vi "LoadFileNew.vi"(11 "folder":string="QAMT01\\CRH3605") -> (1 "f":bool, 3 "Lot":string)   [LabVIEW 2012]
uses:
  Global1.vi
panel:
  out "text":string
  out "before substring":string
  out "after substring":string
  out "String":string
  out "error out":errorcluster
  in  "error in (no error)":errorcluster
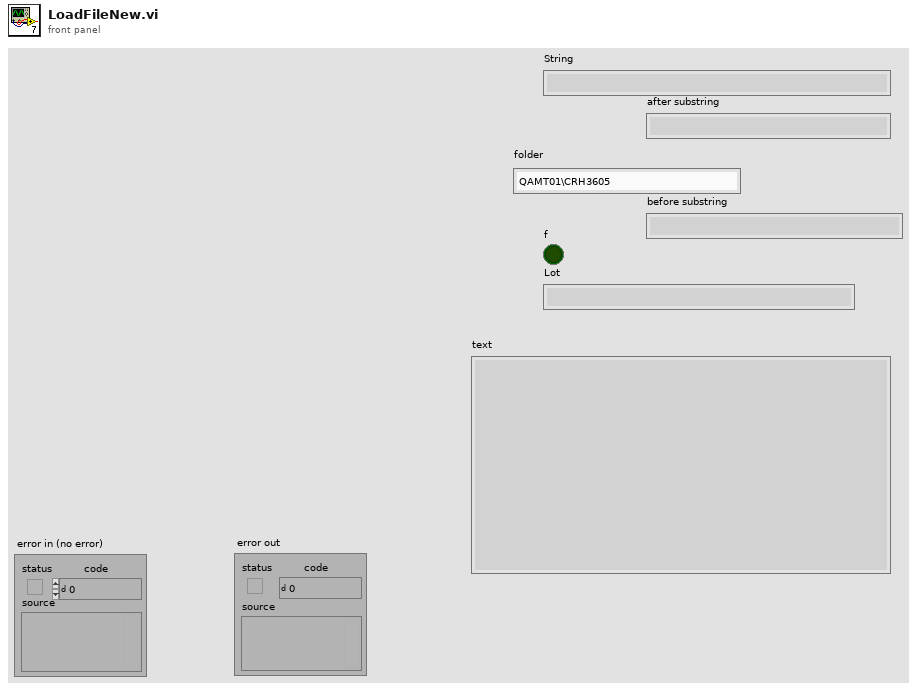
[diagram p1: front panel]
types:
  T1 = enum16{"open", "replace", "create", "open or create", "replace or create", "replace or create with confirmation"}
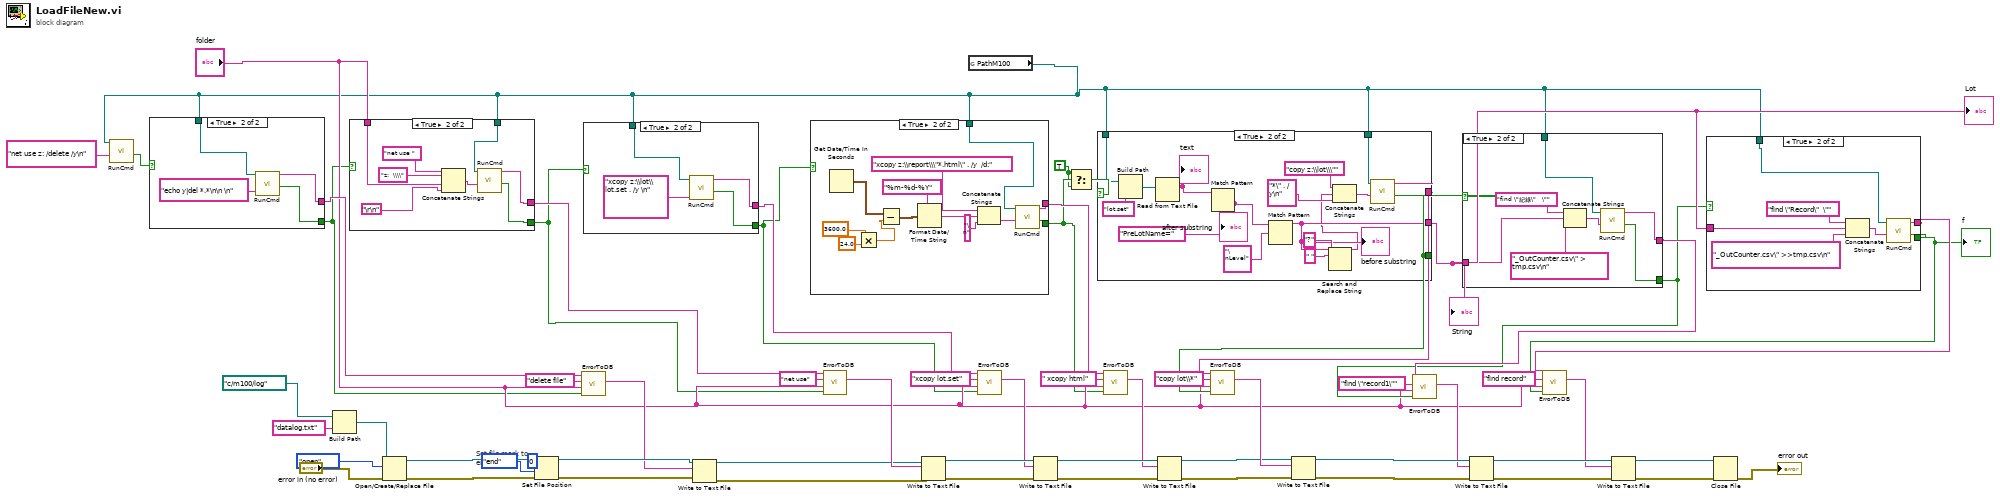
[diagram p0: block diagram]
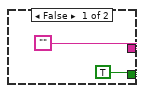
[diagram p2: hidden frame]
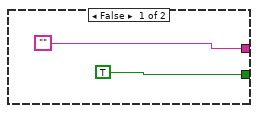
[diagram p3: hidden frame]
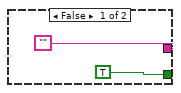
[diagram p4: hidden frame]
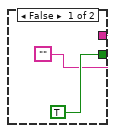
[diagram p5: hidden frame]
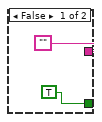
[diagram p6: hidden frame]
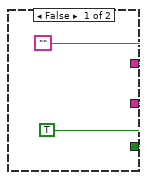
[diagram p7: hidden frame]
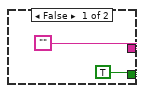
[diagram p8: hidden frame]
diagram:
  w6 = TRUE
  # "Set file mark to\nend of file"
  n1 = Build Path(base path=path "c:/m100/log", name or relative path="datalog.txt") -> (appended path=w53:path)
  n2 = Open/Create/Replace File(file path (use dialog)=w53, error in="error in (no error)", operation (0:open)=T1."open") -> (refnum out=w58:refnum<file>, error out=w57:errorcluster)  [unwired: 3 in, 1 out]
  n3 = Set File Position(offset (in bytes) (0)=i64 0, refnum=w58, from (0:start)=enum16{"start", "end", "current"}."end", error in=w57) -> (refnum out=w22:refnum<file>, error out=w21:errorcluster)
  n4 = global read "Global1.vi" "PathM100"() -> (w5:path)
  n5 = call "RunCmd.vi"("Cmd String"="net use z: /delete /y\n" ("string"), "working directory"=w5) -> ("OK"=w23:bool)  [unwired: 8 in, 1 out]
  n6 = case shown="True" w23 {
    tunnel: [TRUE w65] -> w3
    tunnel: ["" w64] -> w18
    tunnel: w5 -> [_ w67]
    frame False {
    }
    frame True {
      n7 = call "RunCmd.vi"("Cmd String"="echo y|del *.*\n\n \n" ("standard input"), "working directory"=w67) -> ("OK"=w65:bool, "Output"=w64:string)  [unwired: 8 in]
    }
  }
  n8 = case shown="True" w3 {
    tunnel: [TRUE w70] -> w4
    tunnel: ["" w71] -> w31
    tunnel: "folder" -> [_ w73]
    tunnel: w5 -> [_ w72]
    frame False {
    }
    frame True {
      n9 = Concatenate Strings("net use " ("string"), "z:  \\\\" ("string"), w73, "\r\n") -> (w77:string)
      n10 = call "RunCmd.vi"("Cmd String"=w77, "working directory"=w72) -> ("OK"=w70:bool, "Output"=w71:string)  [unwired: 8 in]
    }
  }
  n11 = call "ErrorToDB.vi"("Error"=w3, "Folder"="folder", "Command"="delete file", "Error Message"=w18) -> ("LogData"=w17:string)  [unwired: 7 in]
  n12 = case shown="True" w4 {
    tunnel: [TRUE w81] -> w2
    tunnel: ["" w80] -> w30
    tunnel: w5 -> [_ w83]
    frame False {
    }
    frame True {
      n13 = call "RunCmd.vi"("Cmd String"="xcopy z:\\lot\\lot.set . /y \n" ("standard input"), "working directory"=w83) -> ("OK"=w81:bool, "Output"=w80:string)  [unwired: 8 in]
    }
  }
  n14 = Write to Text File(file (use dialog)=w22, text=w17, error in=w21) -> (refnum out=w20:refnum<file>, error out=w19:errorcluster)  [unwired: 1 in, 1 out]
  n15 = case shown="True" w2 {
    tunnel: [TRUE w87] -> w8
    tunnel: ["" w88] -> w29
    tunnel: w5 -> [_ w86]
    frame False {
    }
    frame True {
      n16 = Get Date/Time In Seconds() -> (seconds since 1Jan1904=w89:timestamp)
      n17 = Multiply(x=3600.0, y=24.0) -> (x*y=w91:dbl)
      n18 = Subtract(x=w89, y=w91) -> (x-y=w92:timestamp)
      n19 = Format Date/Time String(time format string (%c)="%m-%d-%Y", seconds (now)=w92) -> (date/time string=w95:string)  [unwired: 1 in]
      n20 = Concatenate Strings("xcopy z:\\report\\\"*.html\" . /y  /d:" ("string"), w95, "\n" ("string")) -> (w98:string)
      n21 = call "RunCmd.vi"("Cmd String"=w98, "working directory"=w86) -> ("OK"=w87:bool, "Output"=w88:string)  [unwired: 8 in]
    }
  }
  n22 = call "ErrorToDB.vi"("Error"=w4, "Folder"="folder", "Command"="net use", "Error Message"=w31) -> ("LogData"=w43:string)  [unwired: 7 in]
  n23 = Write to Text File(file (use dialog)=w20, text=w43, error in=w19) -> (refnum out=w52:refnum<file>, error out=w51:errorcluster)  [unwired: 1 in, 1 out]
  n24 = call "ErrorToDB.vi"("Error"=w2, "Folder"="folder", "Command"="xcopy lot.set", "Error Message"=w30) -> ("LogData"=w42:string)  [unwired: 7 in]
  n25 = Write to Text File(file (use dialog)=w52, text=w42, error in=w51) -> (refnum out=w28:refnum<file>, error out=w27:errorcluster)  [unwired: 1 in, 1 out]
  n26 = Select(t=w6, s=w8, f=w6) -> (s? t:f=w7:bool)
  n27 = case shown="True" w7 {
    tunnel: [TRUE w105] -> w38
    tunnel: [w99 w106] -> w39
    tunnel: w5 -> [_ w109]
    tunnel: [w99 w102] -> w44
    tunnel: w5 -> [_ w107]
    frame False {
      w99 = ""
    }
    frame True {
      n28 = Build Path(base path=w109, name or relative path="lot.set") -> (appended path=w117:path)
      n29 = Read from Text File(file (use dialog)=w117) -> (text=w114:string)  [unwired: 3 in, 3 out]
      "text" <- w114
      n30 = Match Pattern(string=w114, regular expression="PreLotName=") -> (after substring=w110:string)  [unwired: 1 in, 3 out]
      "after substring" <- w110
      n31 = Match Pattern(string=w110, regular expression="\nLevel") -> (before substring=w102:string)  [unwired: 1 in, 3 out]
      "before substring" <- w102
      n32 = Search and Replace String(input string=w102, search string=" ", replace string="?" ("replace string (\"\")")) -> (result string=w101:string)  [unwired: 5 in, 3 out]
      n33 = Concatenate Strings("copy z:\\lot\\\"" ("string"), w101, "*\" . /y\n" ("string")) -> (w108:string)
      n34 = call "RunCmd.vi"("Cmd String"=w108, "working directory"=w107) -> ("OK"=w105:bool, "Output"=w106:string)  [unwired: 8 in]
    }
  }
  "Lot" <- w44
  "String" <- w44
  n35 = call "ErrorToDB.vi"("Error"=w8, "Folder"="folder", "Command"=" xcopy html", "Error Message"=w29) -> ("LogData"=w24:string)  [unwired: 7 in]
  n36 = Write to Text File(file (use dialog)=w28, text=w24, error in=w27) -> (refnum out=w26:refnum<file>, error out=w25:errorcluster)  [unwired: 1 in, 1 out]
  n37 = call "ErrorToDB.vi"("Error"=w38, "Folder"="folder", "Command"="copy lot\\*", "Error Message"=w39) -> ("LogData"=w40:string)  [unwired: 7 in]
  n38 = Write to Text File(file (use dialog)=w26, text=w40, error in=w25) -> (refnum out=w50:refnum<file>, error out=w49:errorcluster)  [unwired: 1 in, 1 out]
  n39 = case shown="True" w38 {
    tunnel: ["" w121] -> w36
    tunnel: w44 -> [_ w125]
    tunnel: w5 -> [_ w122]
    tunnel: [TRUE w120] -> w35
    frame False {
    }
    frame True {
      n40 = Concatenate Strings("find \"紀錄\"   \"" ("string"), w125, "_OutCounter.csv\" > tmp.csv\n" ("string")) -> (w123:string)
      n41 = call "RunCmd.vi"("Cmd String"=w123, "working directory"=w122) -> ("OK"=w120:bool, "Output"=w121:string)  [unwired: 8 in]
    }
  }
  n42 = call "ErrorToDB.vi"("Error"=w35, "Folder"="folder", "Command"="find \"record1\"", "Error Message"=w36) -> ("LogData"=w37:string)  [unwired: 7 in]
  n43 = Write to Text File(file (use dialog)=w50, text=w37, error in=w49) -> (refnum out=w48:refnum<file>, error out=w46:errorcluster)  [unwired: 1 in, 1 out]
  n44 = case shown="True" w35 {
    tunnel: w5 -> [_ w132]
    tunnel: w44 -> [_ w133]
    tunnel: ["" w129] -> w33
    tunnel: [TRUE w130] -> w32
    frame False {
    }
    frame True {
      n45 = Concatenate Strings("find \"Record\"  \"" ("string"), w133, "_OutCounter.csv\" >>tmp.csv\n" ("string")) -> (w131:string)
      n46 = call "RunCmd.vi"("Cmd String"=w131, "working directory"=w132) -> ("OK"=w130:bool, "Output"=w129:string)  [unwired: 8 in]
    }
  }
  "f" <- w32
  n47 = call "ErrorToDB.vi"("Error"=w32, "Folder"="folder", "Command"="find record", "Error Message"=w33) -> ("LogData"=w34:string)  [unwired: 7 in]
  n48 = Write to Text File(file (use dialog)=w48, text=w34, error in=w46) -> (refnum out=w47:refnum<file>, error out=w45:errorcluster)  [unwired: 1 in, 1 out]
  n49 = Close File(refnum=w47, error in=w45) -> (error out=→"error out":errorcluster)  [unwired: 1 out]
